vi "readini1.vi"(4 "error in (no error)":errorcluster, 5 "Cluster":T1, 6 "section":string="splash.vi", 7 "configuration file path":path=path "C:/skill/7_1/splash/splash.ini") -> (0 "error out":errorcluster, 1 "Dev_Gr":cluster{"DevNo":i32, "Group":string}[](array[cluster]), 2 "global2vi_ref":refnum<vi>, 3 "file path":path)   [LabVIEW 2010]
uses:
  Global 2.vi
  <vilib>/Utility/config.llb/Read Key (I32).vi
  <vilib>/Utility/config.llb/Write Key (I32).vi
  <vilib>/Utility/config.llb/Read Key (String).vi
  <vilib>/Utility/config.llb/Write Key (String).vi
  <vilib>/Utility/config.llb/NI_LVConfig.lvlib
panel:
  out "Array":string[][](array[string]) caption="что читать из файла"
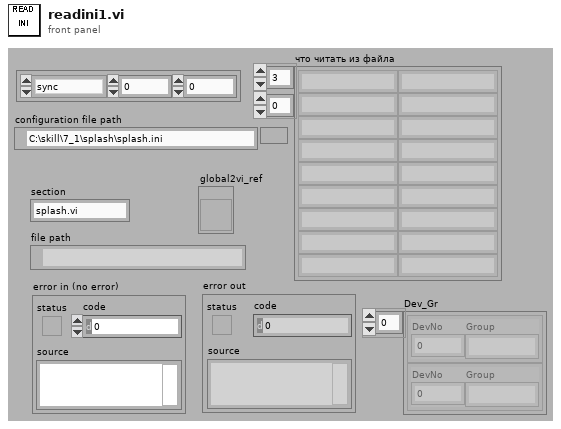
[diagram p1: front panel]
types:
  T1 = cluster{"name":enum16{"sync", "phase_a", "phase_b", "phase_c", "ground"}, "num":i32, "num 2":i32}
  T2 = typedef "NI_LVConfig.lvlib/Config Data RefNum.ctl" = refnum<k1>
  T3 = cluster{"name":enum16{"sync", "phase_a", "phase_b", "phase_c", "ground"}, "num":i32, "num 2":i32}[]
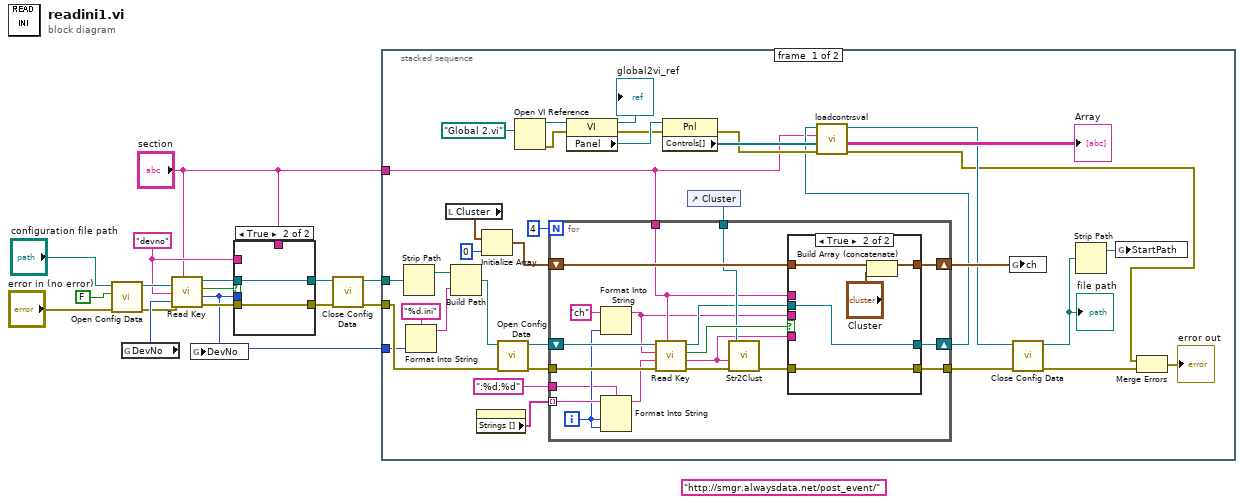
[diagram p0: block diagram]
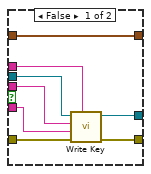
[diagram p2: hidden frame]
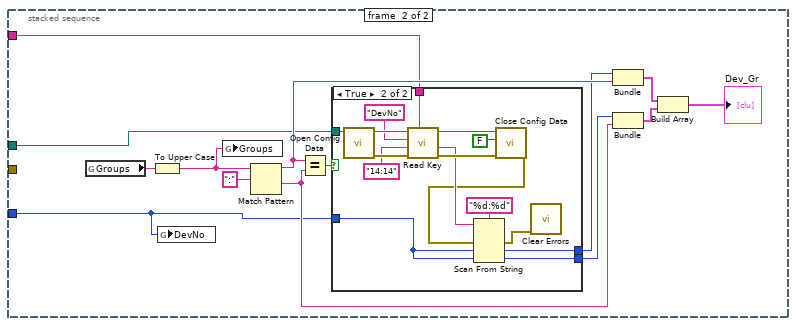
[diagram p3: hidden frame]
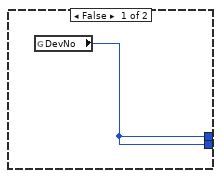
[diagram p4: hidden frame]
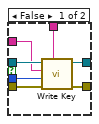
[diagram p5: hidden frame]
diagram:
  w4 = "devno"
  (unwired) "http://smgr.alwaysdata.net/post_event/" ("URL")
  n1 = call <vilib>:"Open Config Data.vi"("error in (no error)"="error in (no error)", "create file if necessary (T)"=FALSE, "configuration file path"="configuration file path") -> ("error out"=w14:errorcluster, "refnum"=w15:T2)  [unwired: 6 in, 1 out]
  n2 = global read "Global 2.vi" "DevNo"() -> (w16:i32)
  n3 = call-poly <vilib>:"Read Key.vi"("section"="section", "error in (no error)"=w14, "default value"=w16, "key"=w4, "refnum"=w15) -> ("error out"=w8:errorcluster, "value"=w5:i32, "found?"=w3:bool, "refnum out"=w9:T2)  [unwired: 3 in]
  n4 = global write "Global 2.vi" "DevNo"(w5) -> ()
  n5 = case shown="True" w3 {
    tunnel: w9 -> [w23 w25]
    tunnel: w8 -> [w22 w24]
    tunnel: "section" -> [w21 _]
    tunnel: [w20 w24] -> w7
    tunnel: [w19 w25] -> w6
    tunnel: w5 -> [w18 _]
    tunnel: w4 -> [w17 _]
    frame False {
      n6 = call-poly <vilib>:"Write Key.vi"("section"=w21, "error in (no error)"=w22, "value"=w18, "key"=w17, "refnum"=w23) -> ("error out"=w20:errorcluster, "refnum out"=w19:T2)  [unwired: 4 in, 1 out]
    }
    frame True {
    }
  }
  n7 = call <vilib>:"Close Config Data.vi"("error in (no error)"=w7, "refnum"=w6) -> ("error out"=w10:errorcluster, "file path"=w2:path)  [unwired: 8 in]
  n8 = stacked-sequence {
    tunnel: w10 -> [w38 _]
    tunnel: w5 -> [w34 w94]
    tunnel: w2 -> [w27 w97]
    tunnel: "section" -> [w26 w96]
    frame #0 {
      n9 = Strip Path(path=w27) -> (stripped path=w42:path)  [unwired: 1 out]
      n10 = Format Into String(format string="%d.ini", w34) -> (resulting string=w40:string)  [unwired: 2 in, 1 out]
      n11 = local read "Cluster"() -> (w37:T1)
      n12 = Build Path(base path=w42, name or relative path=w40) -> (appended path=w41:path)
      n13 = property on="name" class="Enum (strict)"() -> ("Strings []"=w33:string[])  [unwired: 2 in, 2 out]
      n14 = Initialize Array(w37, 0 ("dimension size")) -> (w36:T3)
      n15 = call <vilib>:"Open Config Data.vi"("error in (no error)"=w38, "configuration file path"=w41) -> ("error out"=w43:errorcluster, "refnum"=w44:T2)  [unwired: 7 in, 1 out]
      n16 = Open VI Reference(vi path=path "Global 2.vi") -> (vi reference=w56:refnum<vi>, error out=w55:errorcluster)  [unwired: 5 in]
      n17 = property class="VI"(reference=w56, error in=w55) -> (reference out=→"global2vi_ref":refnum<vi>, error out=w53:errorcluster, "Panel"=w54:refnum<vi>)
      n18 = property class="Pnl"(reference=w54, error in=w53) -> (error out=w48:errorcluster, "Controls[]"=w49:refnum<vi>[])  [unwired: 1 out]
      n19 = control-ref of="Cluster"() -> (w60:refnum<vi>)
      n20 = for {
        N: 4 -> [_]
        tunnel: w43 -> [w79]
        shift-right: [w76] -> w59
        shift-left: w36 -> [w75]
        tunnel: w60 -> [w72]
        tunnel: [w66] -> w58
        shift-right: [w64] -> w47
        shift-left: w44 -> [w78]
        tunnel: w26 -> [w63]
        tunnel: w33 -> [w70] mode=indexing
        tunnel: ":%d:%d" ("key") -> [w67]
        i -> [w69]
        n21 = Format Into String(initial string="ch", w69) -> (resulting string=w61:string)  [unwired: 2 in, 1 out]
        n22 = Format Into String(format string=w67, initial string=w70, w69, w69) -> (resulting string=w68:string)  [unwired: 1 in, 1 out]
        n23 = call-poly <vilib>:"Read Key.vi"("section"=w63, "error in (no error)"=w79, "default value"=w68, "key"=w61, "refnum"=w78) -> ("error out"=w73:errorcluster, "value"=w62:string, "found?"=w74:bool, "refnum out"=w65:T2)  [unwired: 3 in]
        n24 = call "Str2Clust.vi"("error in (no error)"=w73, "String"=w62, "Clust Refnum"=w72) -> ("error out"=w71:errorcluster)  [unwired: 4 in]
        n25 = case shown="True" w74 {
          tunnel: [w87 w92] -> w76
          tunnel: w75 -> [w87 w91]
          tunnel: w71 -> [w86 w89]
          tunnel: [w85 w89] -> w66
          tunnel: w65 -> [w84 w88]
          tunnel: [w83 w88] -> w64
          tunnel: w63 -> [w82 _]
          tunnel: w62 -> [w81 _]
          tunnel: w61 -> [w80 _]
          frame False {
            n26 = call-poly <vilib>:"Write Key.vi"("section"=w82, "error in (no error)"=w86, "value"=w81, "key"=w80, "refnum"=w84) -> ("error out"=w85:errorcluster, "refnum out"=w83:T2)  [unwired: 4 in, 1 out]
          }
          frame True {
            n27 = Build Array (concatenate)(w91, "Cluster") -> (w92:T3)
          }
        }
      }
      n28 = call "loadcontrsval.vi"("error in"=w48, "Array"=w49, "Section"=w26, "refnum in"=w47) -> ("error out"=w29:errorcluster, "Array 2"=→"Array":string[][], "refnum out"=w45:T2)  [unwired: 1 in]
      n29 = global write "Global 2.vi" "ch"(w59) -> ()
      n30 = call <vilib>:"Close Config Data.vi"("error in (no error)"=w58, "refnum"=w45) -> ("error out"=w30:errorcluster, "file path"=w51:path)  [unwired: 8 in]
      "file path" <- w51
      n31 = Strip Path(path=w51) -> (stripped path=w50:path)  [unwired: 1 out]
      n32 = global write "Global 2.vi" "StartPath"(w50) -> ()
      n33 = Merge Errors(w29, w30) -> (→"error out":errorcluster)
    }
    frame #1 {
      n34 = global read "Global 2.vi" "Groups"() -> (w99:string)
      n35 = To Upper Case(1:w99) -> (0:w93:string)
      n36 = global write "Global 2.vi" "DevNo"(w94) -> ()
      n37 = global write "Global 2.vi" "Groups"(w93) -> ()
      n38 = Match Pattern(string=w93, regular expression=":" ("format string")) -> (before substring=w103:string, after substring=w104:string)  [unwired: 1 in, 2 out]
      n39 = Equal?(x=w103, y=w104) -> (x = y?=w100:bool)
      n40 = case shown="True" w100 {
        tunnel: w97 -> [_ w123]
        tunnel: w96 -> [_ w116]
        tunnel: [w107 w112] -> w102
        tunnel: [w107 w111] -> w101
        tunnel: w94 -> [_ w109]
        frame False {
          n41 = global read "Global 2.vi" "DevNo"() -> (w107:i32)
        }
        frame True {
          n42 = call <vilib>:"Open Config Data.vi"("configuration file path"=w123) -> ("error out"=w122:errorcluster, "refnum"=w118:T2)  [unwired: 8 in, 1 out]
          n43 = call-poly <vilib>:"Read Key.vi"("section"=w116, "error in (no error)"=w122, "default value"="14:14", "key"="DevNo", "refnum"=w118) -> ("error out"=w121:errorcluster, "value"=w114:string, "refnum out"=w119:T2)  [unwired: 3 in, 1 out]
          n44 = call <vilib>:"Close Config Data.vi"("error in (no error)"=w121, "write file if changed (T)"=FALSE, "refnum"=w119) -> ("error out"=w110:errorcluster)  [unwired: 7 in, 1 out]
          n45 = Scan From String(format string="%d:%d", input string=w114, error in=w110, default 1=w109, default 2=w109) -> (error out=w108:errorcluster, output 1=w111:i32, output 2=w112:i32)  [unwired: 1 in, 2 out]
          n46 = call <vilib>:"Clear Errors.vi"("error in (no error)"=w108) -> ()  [unwired: 6 in, 1 out]
        }
      }
      n47 = Bundle("value"=w101, w103) -> (w106:cluster{"value":i32, string})  [unwired: 1 in]
      n48 = Bundle("value"=w102, w104) -> (w105:cluster{"value":i32, string})  [unwired: 1 in]
      n49 = Build Array(w106, w105) -> (→"Dev_Gr":cluster{"value":i32, string}[])
    }
  }
